vi "Obtain list values.vi"(8 "error in (no error)":errorcluster, 10 "index (row)":i32, 11 "Soda_Actor in":refnum<class "Soda_Actor.lvclass">) -> (0 "error out":errorcluster, 3 "Soda_Actor out":refnum<class "Soda_Actor.lvclass">)   [LabVIEW 2019, in "Soda_Actor.lvlib" / "Soda_Actor.lvclass"]
uses:
  Soda_Actor.lvclass
  C:/Program Files/National Instruments/LabVIEW 2019/vi.lib/ActorFramework/Actor/Actor.lvclass
  <vilib>/ActorFramework/Actor/Actor.lvclass/Actor.ctl
  Soda_Actor.lvclass/Soda_Actor.ctl
  UI Actor Messages/Update_buy_values Msg/Update_buy_values Msg.lvclass/Update_buy_values Msg.ctl
  <vilib>/ActorFramework/Message Enqueuer/Message Enqueuer.lvclass/Message Enqueuer.ctl
  <vilib>/ActorFramework/Message Enqueuer/Enqueue.vi
  UI Actor Messages/Update_buy_values Msg/Update_buy_values Msg.lvclass
  C:/Program Files/National Instruments/LabVIEW 2019/vi.lib/ActorFramework/Message/Message.lvclass
  <vilib>/ActorFramework/Message Priority Queue/Priority Enqueue.vi
  <vilib>/ActorFramework/Actor/Actor.lvclass
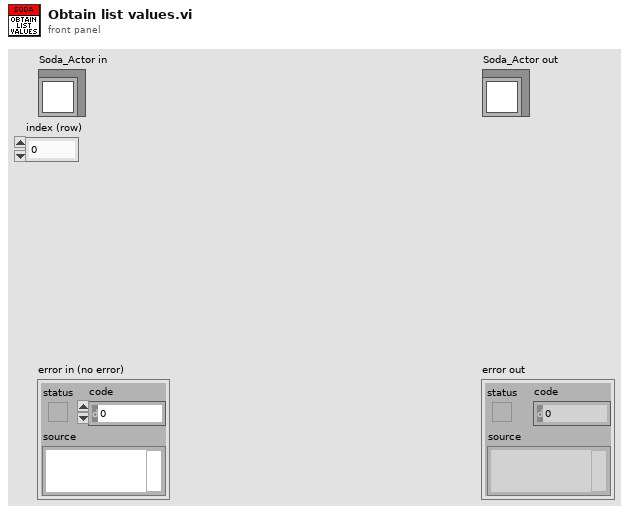
[diagram p1: front panel]
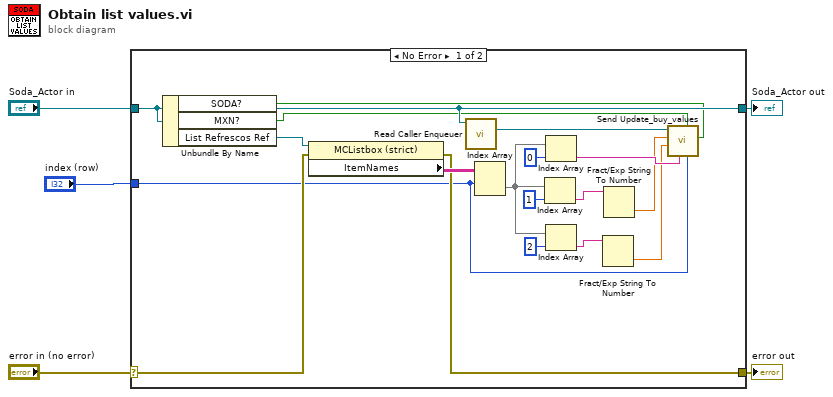
[diagram p0: block diagram]
diagram:
  n1 = case shown="No Error" "error in (no error)" {
    selector: "error in (no error)" -> [w15 w25]
    tunnel: [w14 w25] -> w4
    tunnel: [w10 w24] -> w2
    tunnel: "Soda_Actor in" -> [w10 w24]
    tunnel: "index (row)" -> [w7 _]
    frame No Error {
      n2 = Unbundle By Name(w10) -> ("SODA?"=w6:bool, "MXN?"=w8:bool, "List Refrescos Ref"=w23:refnum<vi>)
      n3 = property class="MCListbox (strict)"(reference=w23, error in=w15) -> (error out=w14:errorcluster, "ItemNames"=w22:string[][])  [unwired: 1 out]
      n4 = call <vilib>:"Read Caller Enqueuer.vi"("Actor"=w10) -> ("Caller Enqueuer"=w9:refnum<class "Message Enqueuer.lvclass">)  [unwired: 10 in]
      n5 = Index Array(array=w22, index (row)=w7) -> (element=w21:string[])  [unwired: 1 in]
      n6 = Index Array(array=w21, index=1) -> (element=w17:string)
      n7 = Index Array(array=w21, index=0) -> (element=w13:string)
      n8 = Index Array(array=w21, index=2) -> (element=w16:string)
      n9 = Fract/Exp String To Number(string=w16) -> (number=w12:dbl)  [unwired: 3 in, 1 out]
      n10 = Fract/Exp String To Number(string=w17) -> (number=w11:dbl)  [unwired: 3 in, 1 out]
      n11 = call "Send Update_buy_values.vi"("SODA?"=w6, "Index"=w7, "MXN?"=w8, "Producto"=w13, "Cantidad"=w12, "Precio"=w11, "Message Enqueuer"=w9) -> ()  [unwired: 3 in, 2 out]
    }
    frame Error {
    }
  }
  "error out" <- w4
  "Soda_Actor out" <- w2
